vi "Read DBC Functions FGV.vi"(7 "Enum":T1=enum."Set Data", 8 "error in (no error)":errorcluster, 11 "DBC FUNCTIONS IN":string[](array[string])) -> (0 "error out":errorcluster, 3 "DBC FUNCTIONS OUT":string[](array[string]))   [LabVIEW 2018]
uses:
  Read File Data.ctl
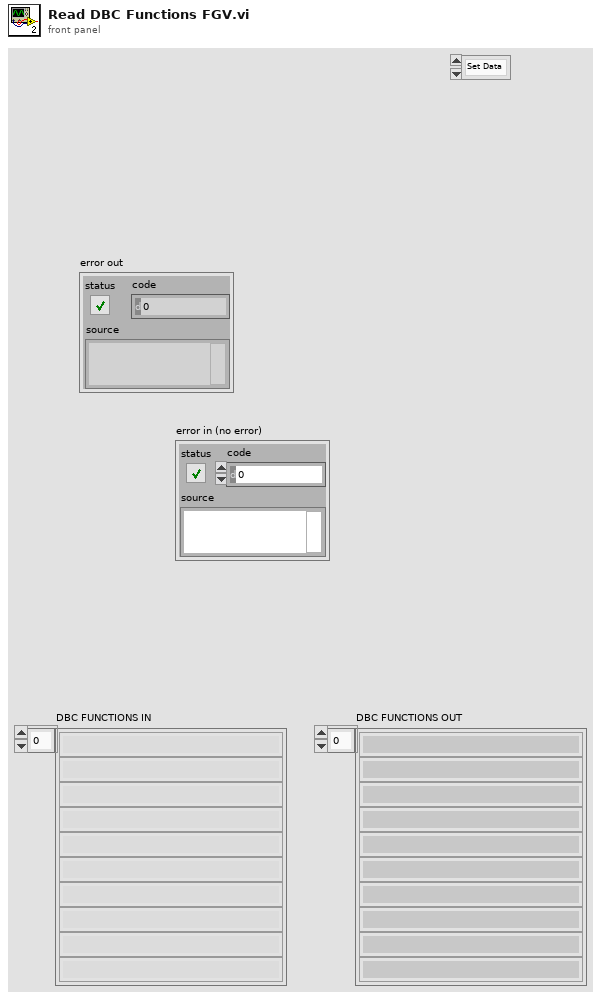
[diagram p1: front panel]
types:
  T1 = typedef "Read File Data.ctl" = enum16{"Get Data", "Set Data"}
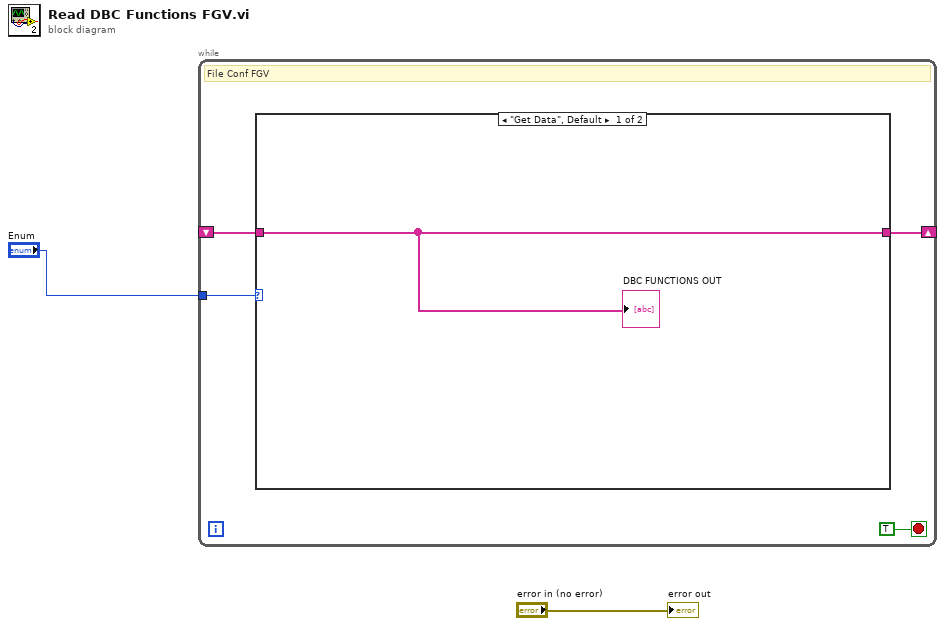
[diagram p0: block diagram]
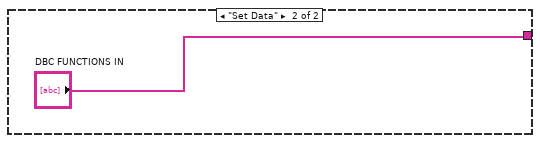
[diagram p2: hidden frame]
diagram:
  n1 = while {
    shift-right: [w5] -> _
    shift-left: _ -> [w4]
    tunnel: "Enum" -> [w3]
    stop <- TRUE stop-if-true
    # "File Conf FGV"
    n2 = case shown="\"Get Data\", Default" w3 {
      tunnel: [w7 "DBC FUNCTIONS IN"] -> w5
      tunnel: w4 -> [w7 _]
      frame "Get Data", Default {
        "DBC FUNCTIONS OUT" <- w7
      }
      frame "Set Data" {
      }
    }
  }
  "error out" <- "error in (no error)"
